vi "Switch Sides.vi"(10 "Lado":enum16{"Esquerdo", "Direito"}(ring) caption="Enum", 11 "Field State Input":T1 {"Detection Frame Out"."robots_blue"."height" format="%+4.3f"; "Detection Frame Out"."robots_blue"."pixel_y" format="%+4.3f"; "Detection Frame Out"."robots_blue"."pixel_x" format="%+4.3f"; "Detection Frame Out"."robots_blue"."orientation" format="%+4.3f"; "Detection Frame Out"."robots_blue"."y" format="%+4.3f"; "Detection Frame Out"."robots_blue"."confidence" format="%4.3f"; "Detection Frame Out"."robots_blue"."x" format="%+4.3f"; "Detection Frame Out"."robots_yellow"."height" format="%+4.3f"; "Detection Frame Out"."robots_yellow"."pixel_y" format="%+4.3f"; "Detection Frame Out"."robots_yellow"."pixel_x" format="%+4.3f"; "Detection Frame Out"."robots_yellow"."orientation" format="%+4.3f"; "Detection Frame Out"."robots_yellow"."y" format="%+4.3f"; "Detection Frame Out"."robots_yellow"."confidence" format="%4.3f"; "Detection Frame Out"."robots_yellow"."x" format="%+4.3f"}) -> (3 "Field State Side Mirrored":T1 {"Detection Frame Out"."robots_blue"."height" format="%+4.3f"; "Detection Frame Out"."robots_blue"."pixel_y" format="%+4.3f"; "Detection Frame Out"."robots_blue"."pixel_x" format="%+4.3f"; "Detection Frame Out"."robots_blue"."orientation" format="%+4.3f"; "Detection Frame Out"."robots_blue"."y" format="%+4.3f"; "Detection Frame Out"."robots_blue"."confidence" format="%4.3f"; "Detection Frame Out"."robots_blue"."x" format="%+4.3f"; "Detection Frame Out"."robots_yellow"."height" format="%+4.3f"; "Detection Frame Out"."robots_yellow"."pixel_y" format="%+4.3f"; "Detection Frame Out"."robots_yellow"."pixel_x" format="%+4.3f"; "Detection Frame Out"."robots_yellow"."orientation" format="%+4.3f"; "Detection Frame Out"."robots_yellow"."y" format="%+4.3f"; "Detection Frame Out"."robots_yellow"."confidence" format="%4.3f"; "Detection Frame Out"."robots_yellow"."x" format="%+4.3f"})   [LabVIEW 2017]
uses:
  <vilib>/Analysis/NI_AAL_Angle.lvlib
  <vilib>/Analysis/coordinate.llb/Wrap Angle (scalar).vi
  SSL Detection Robot.ctl
  SSL Detection Ball.ctl
  SSL Detection Frame.ctl
  SSL/SSL Field State.ctl
  <vilib>/Analysis/Matrix/Datatypes/RealMatrix.ctl
  <vilib>/Analysis/Matrix/NI_Matrix.lvlib
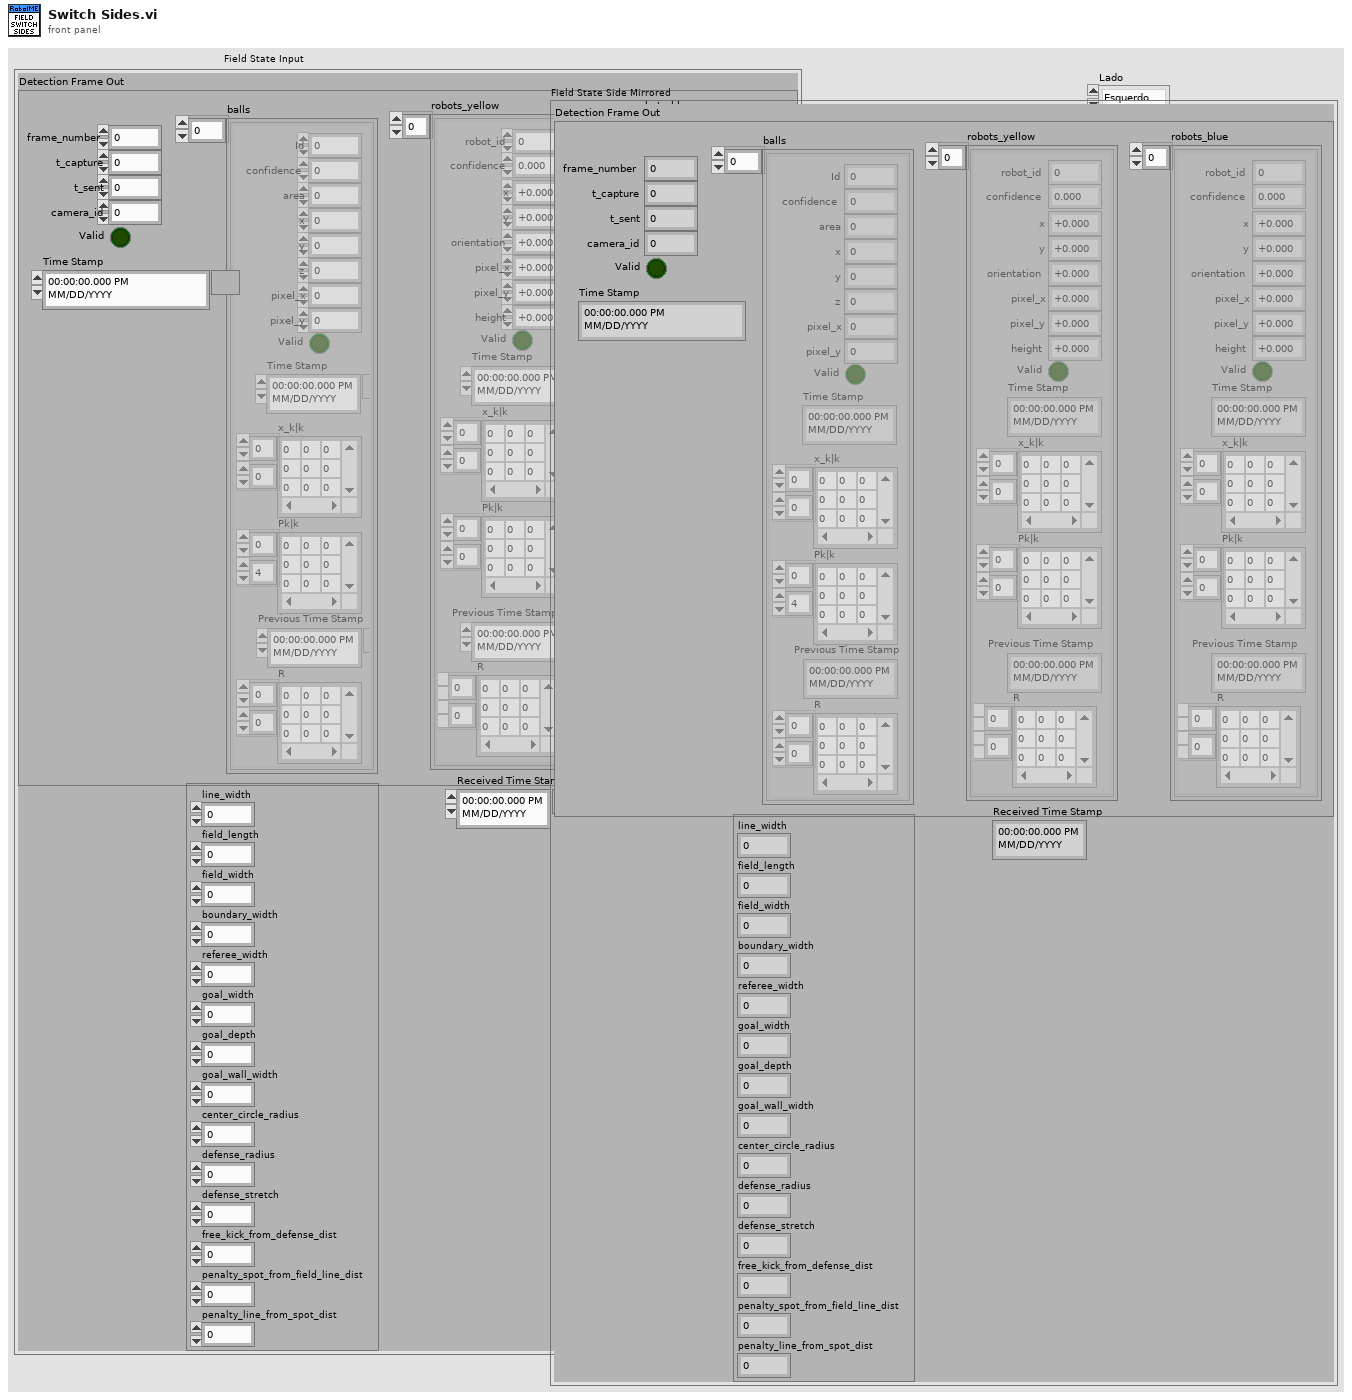
[diagram p1: front panel]
types:
  T1 = typedef "SSL Field State.ctl" = cluster{"Detection Frame Out":T2, "Field Size Out":cluster{"line_width":u32, "field_length":u32, "field_width":u32, "boundary_width":u32, "referee_width":u32, "goal_width":u32, "goal_depth":u32, "goal_wall_width":u32, "center_circle_radius":u32, "defense_radius":u32, "defense_stretch":u32, "free_kick_from_defense_dist":u32, "penalty_spot_from_field_line_dist":u32, "penalty_line_from_spot_dist":u32}, "Received Time Stamp":timestamp}
  T2 = typedef "SSL Detection Frame.ctl" = cluster{"frame_number":u32, "t_capture":dbl, "t_sent":dbl, "camera_id":u32, "robots_yellow":T3[], "robots_blue":T3[], "balls":T5[], "Valid":bool, "Time Stamp":timestamp}
  T3 = typedef "SSL Detection Robot.ctl" = cluster{"x":sgl, "robot_id":u32, "confidence":sgl, "y":sgl, "orientation":sgl, "pixel_x":sgl, "pixel_y":sgl, "height":sgl, "Valid":bool, "Time Stamp":timestamp, "x_k|k":T4, "Pk|k":T4, "Previous Time Stamp":timestamp, "R":T4}
  T4 = typedef "NI_Matrix.lvlib/RealMatrix.ctl" = dbl[][]
  T5 = typedef "SSL Detection Ball.ctl" = cluster{"x":sgl, "area":u32, "confidence":sgl, "y":sgl, "z":sgl, "pixel_x":sgl, "pixel_y":sgl, "Valid":bool, "Time Stamp":timestamp, "x_k|k":T4, "Pk|k":T4, "Id":u32, "Previous Time Stamp":timestamp, "R":T4}
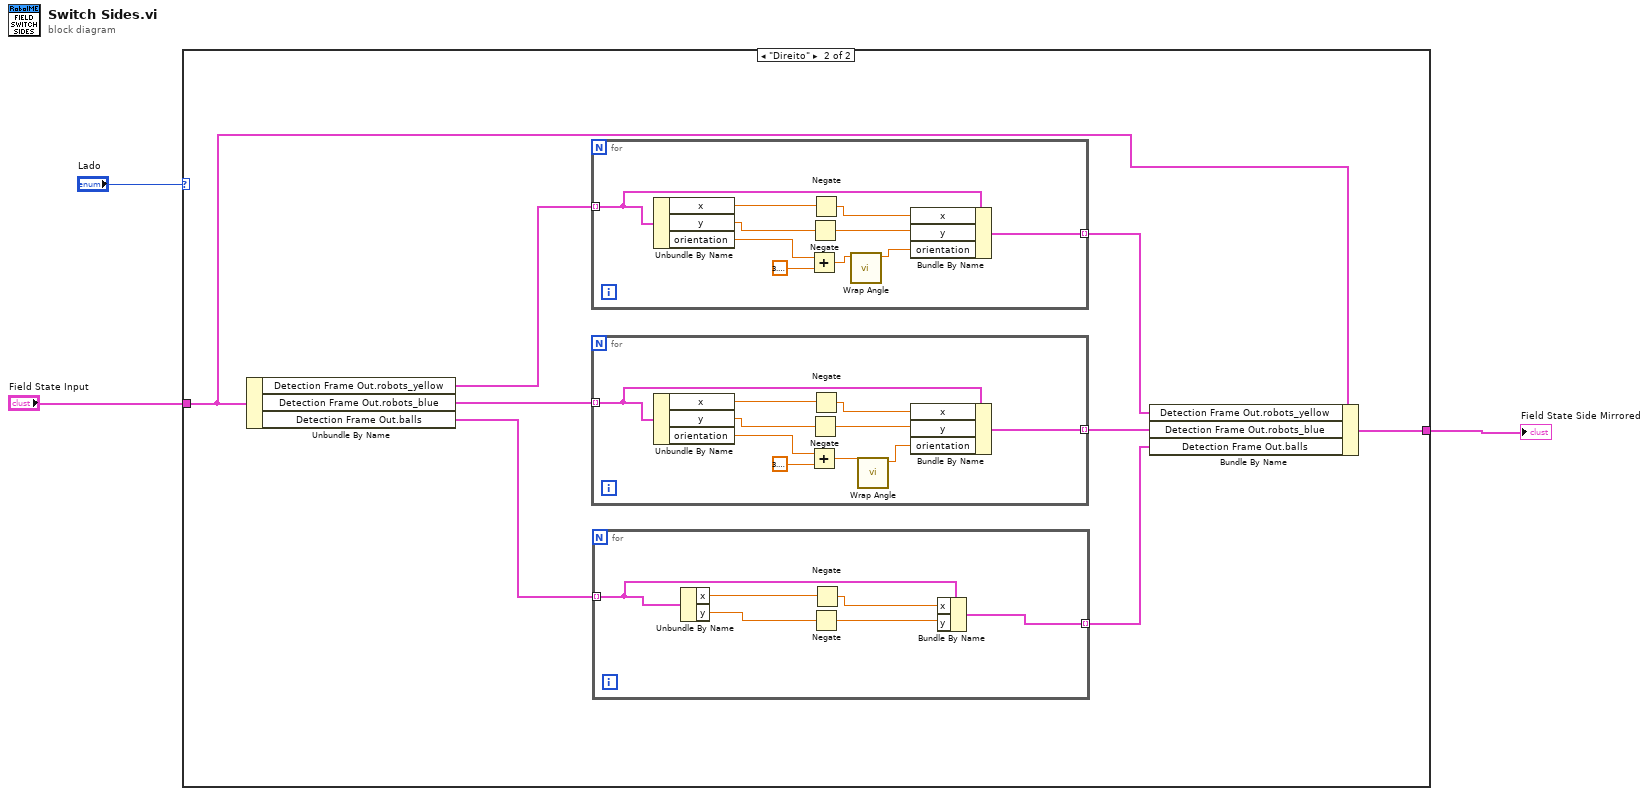
[diagram p0: block diagram]
diagram:
  n1 = case shown="\"Direito\"" "Lado" {
    tunnel: "Field State Input" -> [w4 w6]
    tunnel: [w4 w5] -> w1
    frame "Esquerdo", Default {
    }
    frame "Direito" {
      n2 = Unbundle By Name(w6) -> ("Detection Frame Out.robots_yellow"=w12:T3[], "Detection Frame Out.robots_blue"=w10:T3[], "Detection Frame Out.balls"=w8:T5[])
      n3 = for {
        tunnel: w12 -> [w34] mode=indexing
        tunnel: [w31] -> w11 mode=indexing
        n4 = Unbundle By Name(w34) -> ("x"=w38:sgl, "y"=w37:sgl, "orientation"=w35:sgl)
        n5 = Add(x=w35, y=3.141592653589793) -> (x+y=w30:dbl)
        n6 = Negate(x=w37) -> (-x=w32:sgl)
        n7 = Negate(x=w38) -> (-x=w33:sgl)
        n8 = call-poly <vilib>:"Wrap Angle.vi"("angle in"=w30) -> ("angle out"=w29:dbl)  [unwired: 9 in, 1 out]
        n9 = Bundle By Name(cluster=w34, "x"=w33, "y"=w32, "orientation"=w29) -> (w31:T3)
      }
      n10 = for {
        tunnel: w10 -> [w18] mode=indexing
        tunnel: [w15] -> w9 mode=indexing
        n11 = Unbundle By Name(w18) -> ("x"=w22:sgl, "y"=w21:sgl, "orientation"=w19:sgl)
        n12 = Add(x=w19, y=3.141592653589793) -> (x+y=w14:dbl)
        n13 = Negate(x=w21) -> (-x=w16:sgl)
        n14 = Negate(x=w22) -> (-x=w17:sgl)
        n15 = call-poly <vilib>:"Wrap Angle.vi"("angle in"=w14) -> ("angle out"=w13:dbl)  [unwired: 9 in, 1 out]
        n16 = Bundle By Name(cluster=w18, "x"=w17, "y"=w16, "orientation"=w13) -> (w15:T3)
      }
      n17 = for {
        tunnel: w8 -> [w26] mode=indexing
        tunnel: [w23] -> w7 mode=indexing
        n18 = Unbundle By Name(w26) -> ("x"=w28:sgl, "y"=w27:sgl)
        n19 = Negate(x=w27) -> (-x=w24:sgl)
        n20 = Negate(x=w28) -> (-x=w25:sgl)
        n21 = Bundle By Name(cluster=w26, "x"=w25, "y"=w24) -> (w23:T5)
      }
      n22 = Bundle By Name(cluster=w6, "Detection Frame Out.robots_yellow"=w11, "Detection Frame Out.robots_blue"=w9, "Detection Frame Out.balls"=w7) -> (w5:T1)
    }
  }
  "Field State Side Mirrored" <- w1
